vi "PopulateProbe.vi"(8 "error in (no error)":errorcluster, 10 "Multicolumn Listbox in":refnum<vi>, 11 "LLNode in":refnum<class "LLNode.lvclass">) -> (0 "error out":errorcluster, 2 "Multicolumn Listbox out":refnum<vi>, 3 "LLNode out":refnum<class "LLNode.lvclass">)   [LabVIEW 2009, in "LLNode.lvclass"]
uses:
  LLNode.lvclass
  Node/Node.lvclass
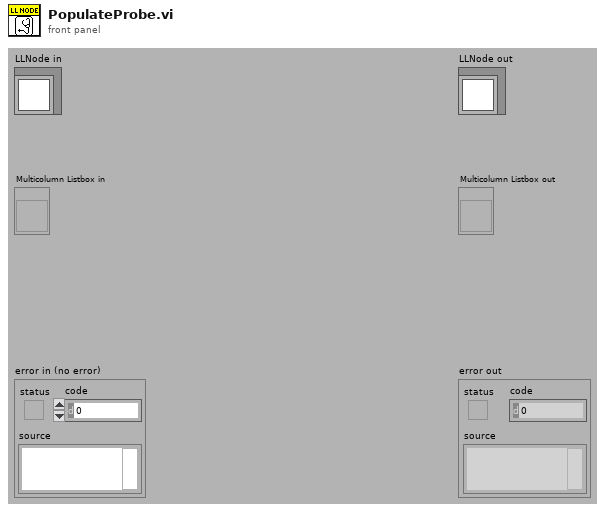
[diagram p1: front panel]
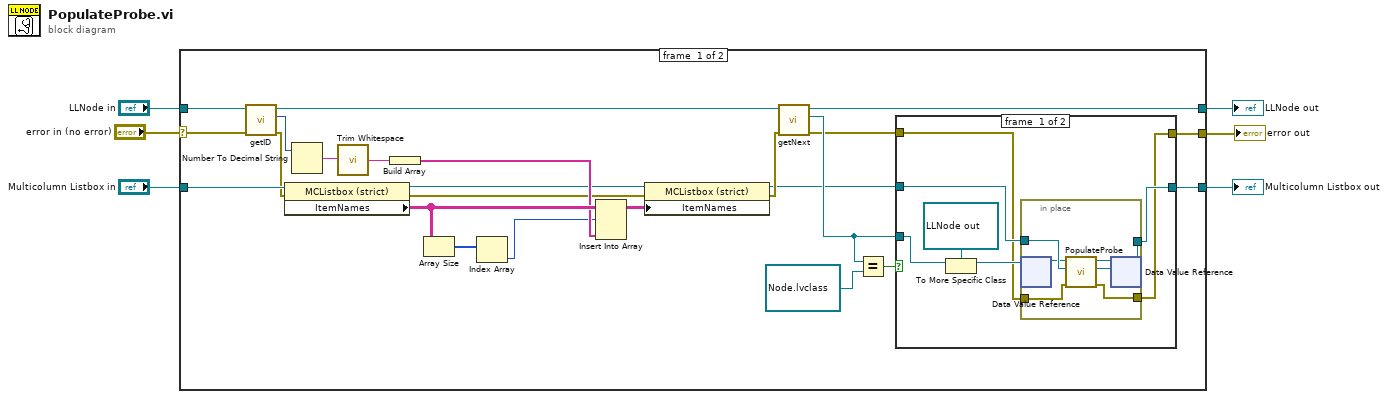
[diagram p0: block diagram]
diagram:
  n1 = case shown="No Error" "error in (no error)" {
    selector: "error in (no error)" -> [w28 w47]
    tunnel: [w14 w48] -> w4
    tunnel: "LLNode in" -> [w30 w48]
    tunnel: "Multicolumn Listbox in" -> [w29 w46]
    tunnel: [w7 w46] -> w2
    tunnel: [w8 w47] -> w1
    frame #0 {
      n2 = call "getID.vi"("error in (no error)"=w28, "Node in"=w30) -> ("error out"=w17:errorcluster, "ID"=w27:u32, "Node out"=w18:refnum<class "LLNode.lvclass">)  [unwired: 7 in]
      n3 = property class="MCListbox (strict)"(reference=w29, error in=w17) -> (reference out=w20:refnum<vi>, error out=w16:errorcluster, "ItemNames"=w24:string[][])
      n4 = Number To Decimal String(number=w27) -> (decimal integer string=w26:string)  [unwired: 1 in]
      n5 = call <vilib>:"Trim Whitespace.vi"("string"=w26) -> ("trimmed string"=w23:string)  [unwired: 1 in]
      n6 = Build Array(w23) -> (w22:string[])
      n7 = Array Size(array=w24) -> (size(s)=w25:i32[])
      n8 = Index Array(array=w25) -> (element=w21:i32)  [unwired: 1 in]
      n9 = Insert Into Array(array=w24, index (row)=w21, new element=w22) -> (w19:string[][])  [unwired: 1 in]
      n10 = property class="MCListbox (strict)"(reference=w20, error in=w16, "ItemNames"=w19) -> (reference out=w10:refnum<vi>, error out=w15:errorcluster)
      n11 = call "getNext.vi"("error in (no error)"=w15, "LLNode in"=w18) -> ("error out"=w9:errorcluster, "next"=w11:refnum<data-value>, "LLNode out"=w14:refnum<class "LLNode.lvclass">)  [unwired: 7 in]
      n12 = Equal?(x=w11, y=refnum<data-value> refnum) -> (x = y?=w12:bool)
      n13 = case shown="True" w12 {
        tunnel: w11 -> [w36 _]
        tunnel: w10 -> [w35 w45]
        tunnel: [w34 w45] -> w7
        tunnel: w9 -> [w32 w44]
        tunnel: [w31 w44] -> w8
        frame #0 {
          n14 = To More Specific Class(target class=refnum<data-value> refnum ("data value reference"), reference=w36) -> (specific class reference=w33:refnum<data-value>)  [unwired: 1 in, 1 out]
          n15 = in-place {
            in-place-border: w35 -> [w43]
            in-place-border: [w42] -> w34
            in-place-border: w32 -> [w39]
            in-place-border: [w38] -> w31
            n16 = in-place-dvr #1(w33) -> (w41:refnum<class "LLNode.lvclass">)  [unwired: 1 out]
            n17 = call-dynamic "PopulateProbe.vi"("error in (no error)"=w39, "Multicolumn Listbox in"=w43, "LLNode in"=w41) -> ("error out"=w38:errorcluster, "Multicolumn Listbox out"=w42:refnum<vi>, "LLNode out"=w40:refnum<class "LLNode.lvclass">)  [unwired: 6 in]
            n18 = in-place-dvr #1(w40) -> ()  [unwired: 2 out]
          }
        }
        frame #1 {
        }
      }
    }
    frame #1 {
    }
  }
  "error out" <- w1
  "LLNode out" <- w4
  "Multicolumn Listbox out" <- w2
